vi "Measure List Measurement Query.vi"(8 "error in":errorcluster, 9 "Meas Number":i32(ring) caption="Measurement Number" items=["Measurement 1", "Measurement 2", "Measurement 3", "Measurement 4", "Measurement 5", "Measurement 6", "Measurement 7", "Measurement 8"], 10 "List Number":i32(ring) items=["List 1", "List 2", "List 3", "List 4"], 11 "Instrument Handle In":i32) -> (0 "error out":errorcluster, 1 "Measurement":i32, 2 "Source":i32, 3 "Instrument Handle Out":i32)   [LabVIEW 8.6, in "ZTScopeM.lvlib"]
doc: "Query the settings of a measurement in a measurement list."
uses:
  ZTScopeM.lvlib
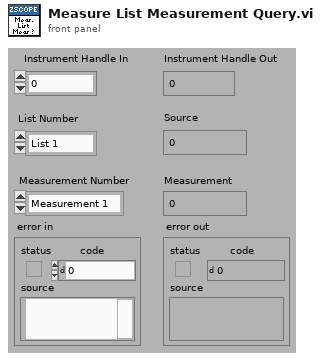
[diagram p1: front panel]
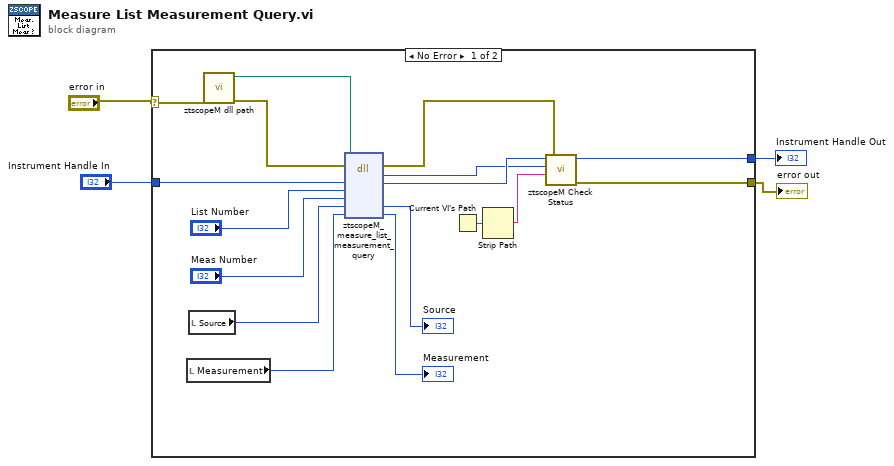
[diagram p0: block diagram]
diagram:
  n1 = case shown="No Error" "error in" {
    selector: "error in" -> [w8 w23]
    tunnel: [w9 w23] -> w1
    tunnel: "Instrument Handle In" -> [w21 w22]
    tunnel: [w10 w22] -> w3
    frame #0 {
      n2 = local read "Measurement"() -> (w16:i32)
      n3 = local read "Source"() -> (w18:i32)
      n4 = call "ztscopeM dll path.vi"("error in (no error)"=w8) -> ("error out"=w6:errorcluster, "<instrument>.dll path"=w7:path)  [unwired: 9 in]
      n5 = dll-call lib="C:/Program Files (x86)/National Instruments/LabVIEW 2013/instr.lib/ztscopem/ztscopeM.dll" fn="ztscopeM_measure_list_measurement_query"(path in=w7, error in=w6, "instrumentHandle"=w21, "listNumber"="List Number", "measurementNumber"="Meas Number", "source"=w18, "Measurement"=w16) -> (error out=w5:errorcluster, w11:i32, "instrumentHandle"=w12:i32, "source"=→"Source":i32, "Measurement"=→"Measurement":i32)  [unwired: 3 in, 1 out]
      n6 = Current VI's Path() -> (path=w14:path)
      n7 = Strip Path(path=w14) -> (name=w13:string)  [unwired: 1 out]
      n8 = call "ztscopeM Check Status.vi"("error in"=w5, "name of VI"=w13, "status (return code)"=w11, "instrument handle in"=w12) -> ("error out"=w9:errorcluster, "instrument handle out"=w10:i32)  [unwired: 2 in]
    }
    frame #1 {
    }
  }
  "Instrument Handle Out" <- w3
  "error out" <- w1
